vi "FIFOStartDAQ_HH.vi"(1 "error in (no error)":errorcluster) -> (0 "error out":errorcluster)   [LabVIEW 2009]
uses:
  hhlib.dll
panel:
  in  "Acq.Time (ms)":i32=1000000
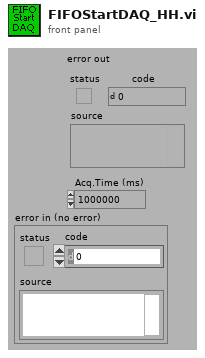
[diagram p1: front panel]
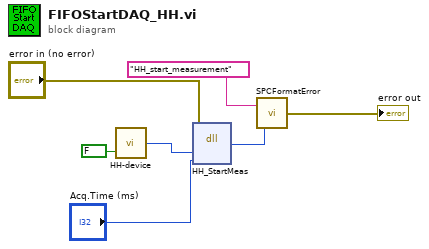
[diagram p0: block diagram]
diagram:
  n1 = call "HH-device.vi"("Set/Get"=FALSE) -> ("Device (output)"=w4:i32)  [unwired: 1 in]
  n2 = dll-call lib="C:/Programme/Anwendungen/DAQLinescan_HH/hhlib.dll" fn="HH_StartMeas" ("SPC_start_measurement")(error in="error in (no error)", "devidx"=w4, "tacq"="Acq.Time (ms)") -> (w6:i32)  [unwired: 4 in, 2 out]
  n3 = call "SPCFormatError.vi"("Error Code"=w6, "Source"="HH_start_measurement") -> ("error out"=→"error out":errorcluster)
